vi "Table-Prevent non-numerics.vi"(8 "error in (no error)":errorcluster, 10 "NewVal in":string[][](array[string]), 11 "OldVal":string[][](array[string])) -> (0 "error out":errorcluster, 2 "Val out":string[][](array[string]), 3 "Discard":bool)   [LabVIEW 2017]
uses:
  <vilib>/Utility/miscctls.llb/LVRowAndColumnTypeDef.ctl
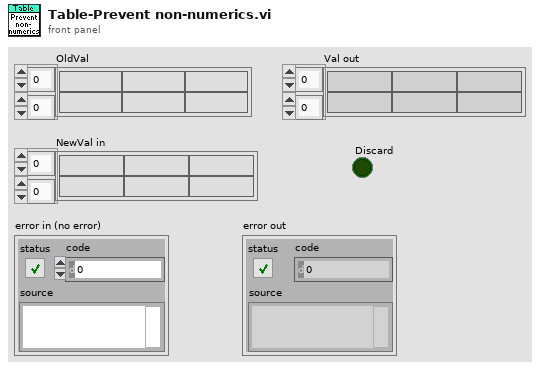
[diagram p1: front panel]
types:
  T1 = typedef "LVRowAndColumnTypeDef.ctl" = cluster{"Row":i32, "Column":i32}
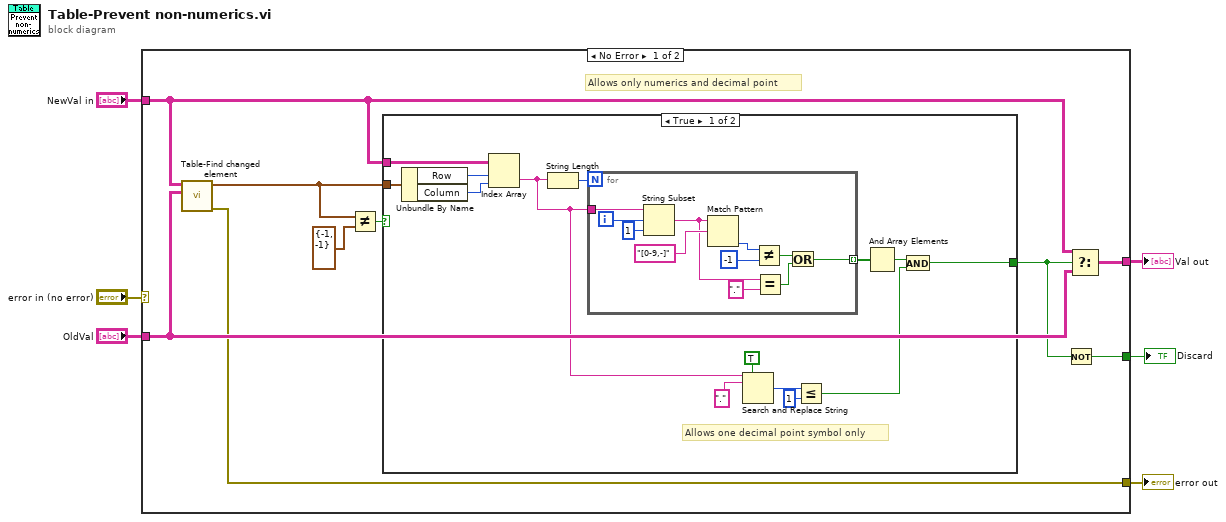
[diagram p0: block diagram]
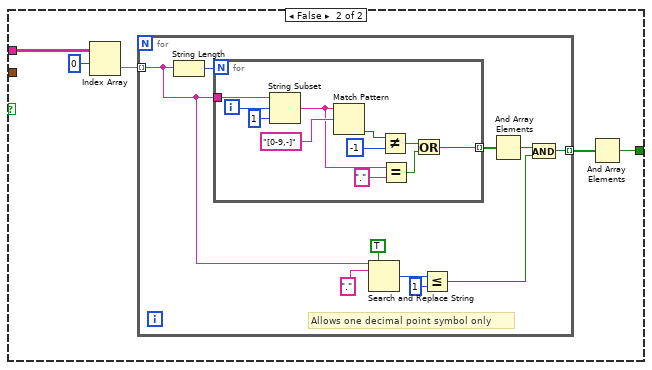
[diagram p2: hidden frame]
diagram:
  n1 = case shown="No Error" "error in (no error)" {
    selector: "error in (no error)" -> [_ w68]
    tunnel: [w15 w67] -> w6
    tunnel: "NewVal in" -> [w8 w67]
    tunnel: "OldVal" -> [w14 _]
    tunnel: [w13 w68] -> w3
    tunnel: [w11 _] -> w1
    frame No Error {
      # "Allows only numerics and decimal point"
      n2 = call "Table-Find changed element.vi"("Table 2"=w14, "Table 1"=w8) -> ("error out"=w13:errorcluster, "Index of change"=w7:T1)  [unwired: 8 in]
      n3 = Not Equal?(x=w7, y=T1 {"Row"=-1, "Column"=-1} ("Index of change")) -> (x != y?=w9:bool)
      n4 = case shown="True" w9 {
        tunnel: [w21 w42] -> w12
        tunnel: w8 -> [w17 w44]
        tunnel: w7 -> [w16 _]
        frame True {
          # "Allows one decimal point symbol only"
          n5 = Unbundle By Name(w16) -> ("Row"=w20:i32, "Column"=w19:i32)
          n6 = Index Array(array=w17, index (row)=w20, index (col)=w19) -> (element=w18:string)
          n7 = String Length(string=w18) -> (length=w29:i32)
          n8 = for {
            N: w29 -> [_]
            tunnel: w18 -> [w40]
            tunnel: [w30] -> w28 mode=indexing
            i -> [w39]
            n9 = String Subset(string=w40, offset (0)=w39, length (rest)=1 ("length (rest)")) -> (substring=w34:string)
            n10 = Match Pattern(string=w34, regular expression="[0-9,-]") -> (offset past match=w36:i32)  [unwired: 1 in, 3 out]
            n11 = Not Equal?(x=w36, y=-1 ("default (0 I32)")) -> (x != y?=w31:bool)
            n12 = Equal?(x=w34, y=".") -> (x = y?=w32:bool)
            n13 = Or(x=w31, y=w32) -> (x .or. y?=w30:bool)
          }
          n14 = Search and Replace String(replace all?=TRUE ("replace all? (F)"), input string=w18, search string="." ("y")) -> (number of replacements=w26:i32)  [unwired: 5 in, 3 out]
          n15 = Less Or Equal?(x=w26, y=1) -> (x <= y?=w23:bool)
          n16 = And Array Elements(Boolean array=w28) -> (logical AND=w24:bool)
          n17 = And(x=w24, y=w23) -> (x .and. y?=w21:bool)
        }
        frame False {
          n18 = Index Array(array=w44, index (row)=0 ("disabled index (row)")) -> (element=w45:string[])  [unwired: 1 in]
          n19 = for {
            tunnel: [w47] -> w41 mode=indexing
            tunnel: w45 -> [w46] mode=indexing
            # "Allows one decimal point symbol only"
            n20 = String Length(string=w46) -> (length=w55:i32)
            n21 = for {
              N: w55 -> [_]
              tunnel: w46 -> [w66]
              tunnel: [w56] -> w54 mode=indexing
              i -> [w65]
              n22 = String Subset(string=w66, offset (0)=w65, length (rest)=1 ("length (rest)")) -> (substring=w60:string)
              n23 = Match Pattern(string=w60, regular expression="[0-9,-]") -> (offset past match=w62:i32)  [unwired: 1 in, 3 out]
              n24 = Not Equal?(x=w62, y=-1 ("default (0 I32)")) -> (x != y?=w57:bool)
              n25 = Equal?(x=w60, y=".") -> (x = y?=w58:bool)
              n26 = Or(x=w57, y=w58) -> (x .or. y?=w56:bool)
            }
            n27 = Search and Replace String(replace all?=TRUE ("replace all? (F)"), input string=w46, search string="." ("y")) -> (number of replacements=w52:i32)  [unwired: 5 in, 3 out]
            n28 = Less Or Equal?(x=w52, y=1) -> (x <= y?=w49:bool)
            n29 = And Array Elements(Boolean array=w54) -> (logical AND=w50:bool)
            n30 = And(x=w50, y=w49) -> (x .and. y?=w47:bool)
          }
          n31 = And Array Elements(Boolean array=w41) -> (logical AND=w42:bool)
        }
      }
      n32 = Not(x=w12) -> (.not. x?=w11:bool)
      n33 = Select(t=w8, s=w12, f=w14) -> (s? t:f=w15:string[][])
    }
    frame Error {
    }
  }
  "Val out" <- w6
  "error out" <- w3
  "Discard" <- w1
